vi "Table Write.vi"(4 "error in (no error)":errorcluster, 5 "Value":variant, 6 "Container State":T6, 7 "Display State In":T1) -> (0 "error out":errorcluster, 3 "Display State Out":T1)   [LabVIEW 2020, in "KTable.xctl"]
uses:
  KTable.xctl
  <vilib>/_xctls/Container State.ctl
  State.ctl
  ColumnSpec.ctl
  ColumnType.ctl
  Table Properties.ctl
  Events.ctl
  Event Data.ctl
  Event Type.ctl
  <vilib>/Utility/miscctls.llb/LVRowAndColumnUnsignedTypeDef.ctl
  Array Manipulation VIs/Array-Dimensions (2D string).vi
  <vilib>/_xctls/XControlSupport.lvlib
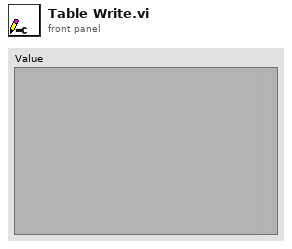
[diagram p1: front panel]
types:
  T1 = typedef "KTable.xctl/State.ctl" = cluster{"Columns":T2[], "Listbox":refnum<vi>, "Default row":string[], "Properties":T4, "Events":T5, "Locked":bool[][], "Size":cluster{"Rows":i32, "Columns":i32}, "rings":i32[][], "DefColors":u32[]}
  T2 = typedef "KTable.xctl/ColumnSpec.ctl" = cluster{"Name":string, "Type":T3, "Width":i32, "Strings":string[], "Position":enum16{"Left", "Center", "Right"}, "locked":bool, "cds":cluster{"Strings":string[]}[][], "Hide NaN":bool}
  T3 = typedef "KTable.xctl/ColumnType.ctl" = enum16{"String", "Enum", "Int", "Double", "Boolean", "Ring", "Formula", "Color"}
  T4 = typedef "KTable.xctl/Table Properties.ctl" = cluster{"Vertical scrollbar":bool, "User add/delete":bool, "Max rows":i32, "Row headers":bool}
  T5 = typedef "KTable.xctl/Events.ctl" = cluster{"Items Changed":refnum<user-event>}
  T6 = typedef "XControlSupport.lvlib/Container State.ctl" = cluster{"Indicator?":bool, "Run Mode?":bool, " Refnum":refnum<vi>}
  T7 = typedef "LVRowAndColumnUnsignedTypeDef.ctl" = cluster{"Row":u32, "Column":u32}
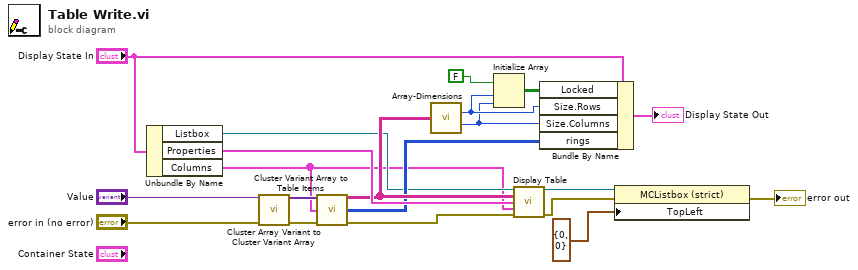
[diagram p0: block diagram]
diagram:
  n1 = Unbundle By Name("Display State In") -> ("Listbox"=w2:refnum<vi>, "Properties"=w15:T4, "Columns"=w1:T2[])
  n2 = call "Cluster Array Variant to Cluster Variant Array.vi"("Variant"="Value", "error in (no error)"="error in (no error)") -> ("Array"=w19:variant[], "error out"=w18:errorcluster)  [unwired: 12 in]
  n3 = call "Cluster Variant Array to Table Items.vi"("Cluster Variant Array"=w19, "Columns"=w1, "error in (no error)"=w18) -> ("Table Items"=w14:string[][], "rings"=w8:i32[][], "error out"=w4:errorcluster)  [unwired: 10 in]
  n4 = call-poly "Array-Dimensions.vi"("2D Array"=w14) -> ("# rows"=w10:i32, "# columns"=w9:i32)  [unwired: 13 in]
  n5 = Initialize Array(FALSE, w10, w9) -> (w11:bool[][])
  n6 = call "Display Table.vi"("Listbox"=w2, "Table Items"=w14, "Properties"=w15, "Columns"=w1, "error in (no error)"=w4) -> ("reference out"=w5:refnum<vi>, "error out"=w7:errorcluster)  [unwired: 9 in]
  n7 = Bundle By Name(cluster="Display State In", "Locked"=w11, "Size.Rows"=w10, "Size.Columns"=w9, "rings"=w8) -> (→"Display State Out":T1)
  n8 = property class="MCListbox (strict)"(reference=w5, error in=w7, "TopLeft"=T7 {"Row"=0, "Column"=0} ("Top Left Visible Cell")) -> (error out=→"error out":errorcluster)  [unwired: 1 out]
